vi "CABLE_SetCuff_Hip.vi"(8 "Hip Cuff Forward Shift (m)":dbl, 9 "Hip Cuff Height (m)":dbl, 10 "Hip Cuff Width (m)":dbl, 11 "Hip Width (m)":dbl) -> (3 "Hip Cuff":T1={"BodyID"=0, "CoM(CuffCS)"={"Coord4"=[0.0, 0.0, 0.0, 1.0], "ID"=0}, "Mass(kg)"=0.0, "CablePts(CuffCS)"=[], "Cuff->Body"=[[1.0, 0.0, 0.0, 0.0], [0.0, 1.0, 0.0, 0.0], [0.0, 0.0, 1.0, 0.0], [0.0, 0.0, 0.0, 1.0]]})   [LabVIEW 2016, in "CAlex2.lvclass"]
uses:
  CAlex2.lvclass
  SerialChain-Cable/TypeDef/Cuff.ctl
  SerialChain/TypeDef/PointOnBody.ctl
  <vilib>/Analysis/Matrix/Datatypes/RealMatrix.ctl
  SerialChain/TypeDef/xyzO.ctl
  SerialChain/SerialChain.lvclass
  <vilib>/Analysis/Matrix/NI_Matrix.lvlib
  SerialChain-Cable/SerialChain-Cable.lvclass
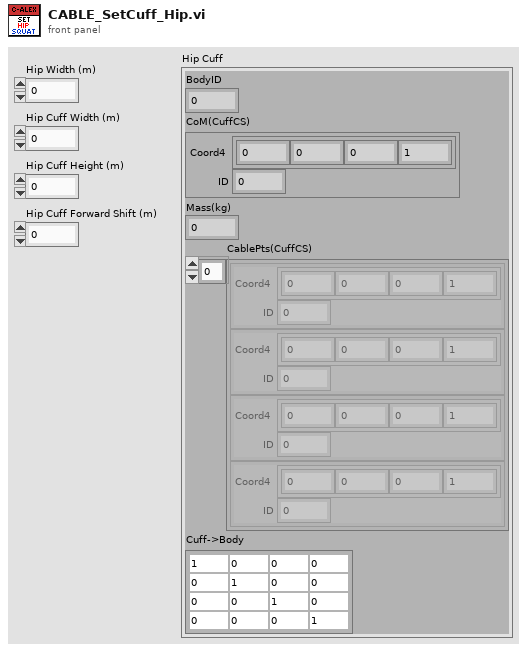
[diagram p1: front panel]
types:
  T1 = typedef "SerialChain-Cable.lvclass/Cuff.ctl" = cluster{"BodyID":i32, "CoM(CuffCS)":T2, "Mass(kg)":dbl, "CablePts(CuffCS)":T2[], "Cuff->Body":T3}
  T2 = typedef "SerialChain.lvclass/PointOnBody.ctl" = cluster{"Coord4":dbl[], "ID":i32}
  T3 = typedef "NI_Matrix.lvlib/RealMatrix.ctl" = dbl[][]
  T4 = typedef "SerialChain.lvclass/xyzO.ctl" = enum16{"X", "Y", "Z", "O"}
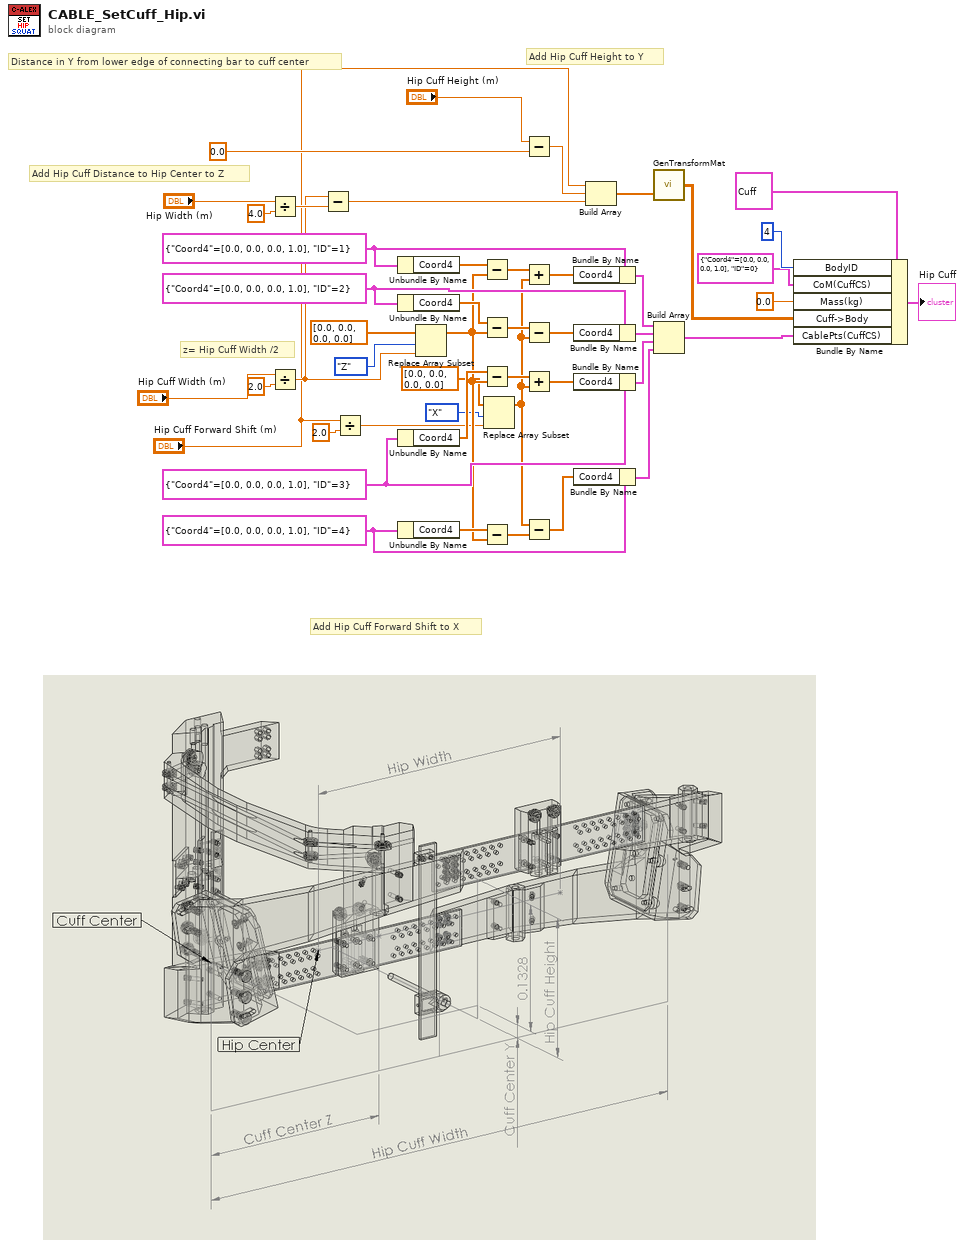
[diagram p0: block diagram]
diagram:
  w26 = T2 {"Coord4"=[0.0, 0.0, 0.0, 1.0], "ID"=1} ("CoM(CuffCS)")
  w25 = T2 {"Coord4"=[0.0, 0.0, 0.0, 1.0], "ID"=2} ("CoM(CuffCS)")
  w14 = T2 {"Coord4"=[0.0, 0.0, 0.0, 1.0], "ID"=4} ("CoM(CuffCS)")
  w17 = T2 {"Coord4"=[0.0, 0.0, 0.0, 1.0], "ID"=3} ("CoM(CuffCS)")
  # "Distance in Y from lower edge of connecting bar to cuff center"
  # "Add Hip Cuff Distance to Hip Center to Z"
  # "Add Hip Cuff Forward Shift to X"
  # "z= Hip Cuff Width /2"
  # "Add Hip Cuff Height to Y"
  n1 = Divide(x="Hip Width (m)", y=4.0) -> (x/y=w30:dbl)
  n2 = Divide(x="Hip Cuff Width (m)", y=2.0) -> (x/y=w29:dbl)
  n3 = Subtract(x=w29, y=w30) -> (x-y=w28:dbl)
  n4 = Divide(x="Hip Cuff Forward Shift (m)", y=2.0) -> (x/y=w8:dbl)
  n5 = Unbundle By Name(w26) -> ("Coord4"=w38:dbl[])
  n6 = Unbundle By Name(w25) -> ("Coord4"=w41:dbl[])
  n7 = Unbundle By Name(w17) -> ("Coord4"=w18:dbl[])
  n8 = Unbundle By Name(w14) -> ("Coord4"=w15:dbl[])
  n9 = Replace Array Subset(array=dbl[] [0.0, 0.0, 0.0, 0.0] ("Coord4"), new element=w29, index=xyzO."Z" ("XYZ")) -> (w11:dbl[])
  n10 = Subtract(x=w38, y=w11) -> (x-y=w42:dbl[])
  n11 = Subtract(x=w41, y=w11) -> (x-y=w43:dbl[])
  n12 = Subtract(x=w18, y=w11) -> (x-y=w19:dbl[])
  n13 = Subtract(x=w15, y=w11) -> (x-y=w16:dbl[])
  n14 = Replace Array Subset(array=dbl[] [0.0, 0.0, 0.0, 0.0] ("Coord4"), new element=w8, index=xyzO."X" ("XYZ")) -> (w1:dbl[])
  n15 = Subtract(x="Hip Cuff Height (m)", y=0.0) -> (x-y=w21:dbl)
  n16 = Add(x=w42, y=w1) -> (x+y=w5:dbl[])
  n17 = Subtract(x=w43, y=w1) -> (x-y=w4:dbl[])
  n18 = Add(x=w19, y=w1) -> (x+y=w3:dbl[])
  n19 = Subtract(x=w1, y=w16) -> (x-y=w2:dbl[])
  n20 = Bundle By Name(cluster=w26, "Coord4"=w5) -> (w36:T2)
  n21 = Bundle By Name(cluster=w25, "Coord4"=w4) -> (w37:T2)
  n22 = Bundle By Name(cluster=w17, "Coord4"=w3) -> (w13:T2)
  n23 = Bundle By Name(cluster=w14, "Coord4"=w2) -> (w12:T2)
  n24 = Build Array("Hip Cuff Forward Shift (m)", w21, w28) -> (w24:dbl[])
  n25 = call "GenTransformMat.vi"("Translate 3Vector"=w24) -> ("Transformation Matrix"=w23:T3)  [unwired: 1 in]
  n26 = Build Array(w36, w37, w13, w12) -> (w35:T2[])
  n27 = Bundle By Name(cluster=T1 {"BodyID"=0, "CoM(CuffCS)"={"Coord4"=[0.0, 0.0, 0.0, 1.0], "ID"=0}, "Mass(kg)"=0.0, "CablePts(CuffCS)"=[], "Cuff->Body"=[[1.0, 0.0, 0.0, 0.0], [0.0, 1.0, 0.0, 0.0], [0.0, 0.0, 1.0, 0.0], [0.0, 0.0, 0.0, 1.0]]} ("Cuff Design"), "BodyID"=4, "CoM(CuffCS)"=T2 {"Coord4"=[0.0, 0.0, 0.0, 1.0], "ID"=0}, "Mass(kg)"=0.0, "Cuff->Body"=w23, "CablePts(CuffCS)"=w35) -> (→"Hip Cuff":T1)
